vi "runTestScenario.vi"(8 "error in (no error)":errorcluster, 11 "SM_CW High Test in":refnum<class "SM_CW High Test.lvclass">) -> (0 "error out":errorcluster, 2 "TestExecution":T1, 3 "SM_CW High Test out":refnum<class "SM_CW High Test.lvclass">)   [LabVIEW 2015, in "SM_CW High Test.lvclass"]
uses:
  SM_CW High Test.lvclass
  Typedefs/TestExecution.ctl
  SM_CW High Test.lvclass/SM_CW High Test.ctl
  <userlib>/Common/ILC/Typedefs/DigitalOutputValues.ctl
  Typedefs/WriteLogMessageInput.ctl
  Typedefs/TestScenarioTypes.ctl
  Typedefs/PassFailTest.ctl
  Model/TestLog/ITestLog/ITestLog.lvclass
  Typedefs/ILCBTTypedefs.lvlib
  <userlib>/Common/ILC/ILC/ILC.lvclass
  <userlib>/Common/ILC/Typedefs/ILCTypedefs.lvlib
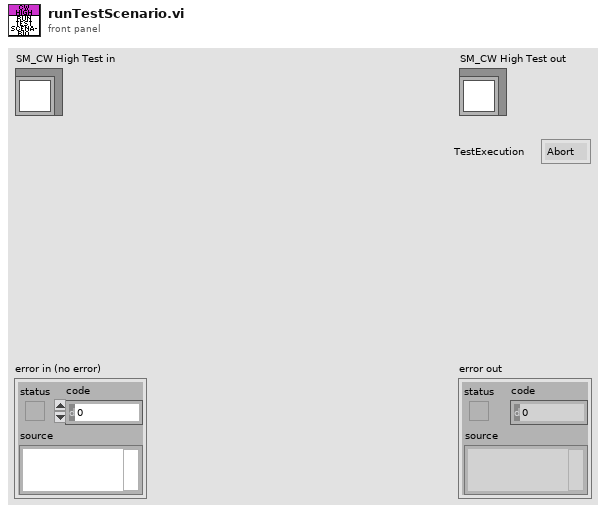
[diagram p1: front panel]
types:
  T1 = typedef "ILCBTTypedefs.lvlib/TestExecution.ctl" = enum16{"Abort", "Continue"}
  T2 = typedef "ILCBTTypedefs.lvlib/Digital Signal Level.ctl" = enum16{"Low", "High"}
  T3 = typedef "ILCBTTypedefs.lvlib/WriteLogMessageInput.ctl" = cluster{"Test Scenario":T4, "Description":string, "Actual Value":string, "Data File":string, "Result":T5}
  T4 = typedef "ILCBTTypedefs.lvlib/TestScenarioTypes.ctl" = enum16{"+3.3VA Supply Test", "+3.3VD Supply Test", "+5VA Supply Test", "+5VD Supply Test", "Unique ID Test", "TEDS Status Test", "LIMSW1_TTL Low Test", "LIMSW1_TTL High Test", "LIMSW2_TTL Low Test", "LIMSW2_TTL High Test", "Tachometer Test", "SSR_TTL Low Test", "SSR_TTL High Test", "SM_CW Low Test", "SM_CW High Test", "SM_CCW Low Test", "SM_CCW High Test", "SM_GPI Low Test", "SM_GPI High Test", "CW Motion Without Limit Test", "CW Motion With Limit Test", "CW Motion With Limit Interruption Test", "CW Motion on CCW Limit Test", "CCW Motion Without Limit Test", "CCW Motion With Limit Test", "CCW Motion With Limit Interruption Test", "CCW Motion on CW Limit Test", "RS232-TXD Low Test", "RS232-TXD High Test", "RS232-RTS Low Test", "RS232-RTS High Test", "RS232-RXD Low Test", "RS232-RXD High Test", "RS232-CTS Low Test", "RS232-CTS High Test", "Out_SS Low Test", "Out_SS High Test", "Out_SDI Low Test", "Out_SDI High Test", "Out_SCLK Low Test", "Out_SCLK High Test", "Reset Low Test", "Reset High Test", "1 Channel ADC Test", "3 Channel ADC Test", "5 Channel ADC Test", "Vref Test", "ROT Test", "DAC1 Test", "DAC2 Test", "DAC3 Test", "DAC4 Test", "BIAS Test", "EXC1 Test", "EXC2 Test", "EXC3 Test", "EXC4 Test"}
  T5 = typedef "ILCBTTypedefs.lvlib/PassFailTest.ctl" = enum16{"Fail", "Pass", "NA"}
  T6 = typedef "ILCCommon.lvlib/ILCTypedefs.lvlib/DigitalOutputValues.ctl" = cluster{"All Off":bool, "SM_CW":bool, "SM_CCW":bool, "UART2_TXD":bool, "UART2_RTS":bool, "UART2_RXD":bool, "UART2_CTS":bool, "OUT_SDO":bool, "OUT_SDI":bool, "OUT_SCK":bool, "MB_SS":bool, "MB_RESET":bool, "SSR_OUT":bool}
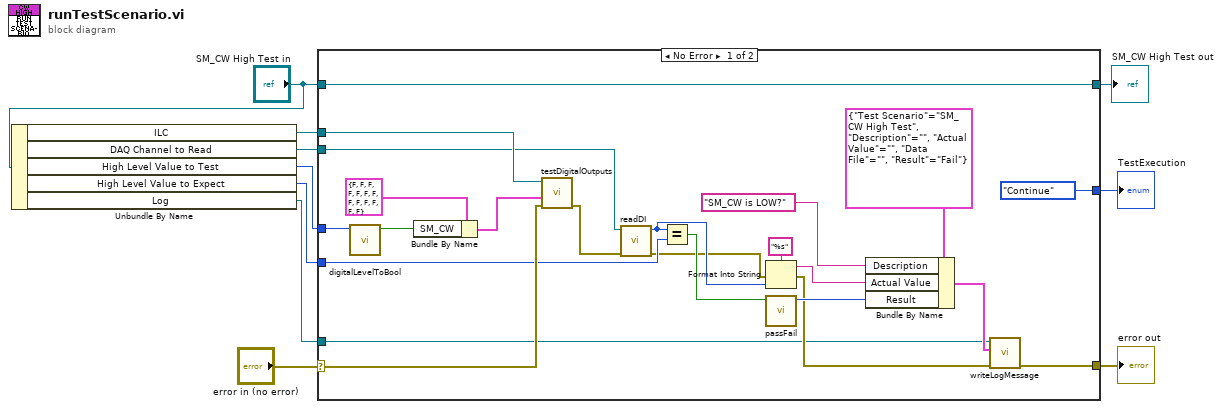
[diagram p0: block diagram]
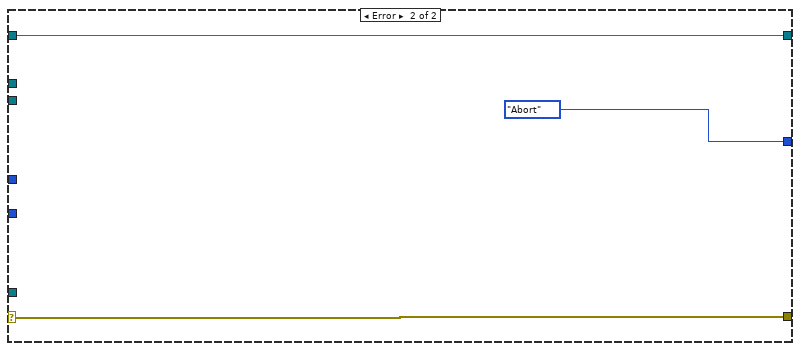
[diagram p2: hidden frame]
diagram:
  n1 = Unbundle By Name("SM_CW High Test in") -> ("ILC"=w4:refnum<class "ILC.lvclass">, "DAQ Channel to Read"=w3:refnum<k21>, "High Level Value to Test"=w5:T2, "High Level Value to Expect"=w2:T2, "Log"=w1:refnum<class "ITestLog.lvclass">)
  n2 = case shown="No Error" "error in (no error)" {
    selector: "error in (no error)" -> [w32 w35]
    tunnel: [w13 w35] -> w9
    tunnel: [w30 w36] -> w8
    tunnel: "SM_CW High Test in" -> [w30 w36]
    tunnel: [TestExecution."Continue" ("TestExecution") TestExecution."Abort" ("TestExecution")] -> w7
    tunnel: w5 -> [w27 _]
    tunnel: w4 -> [w26 _]
    tunnel: w3 -> [w24 _]
    tunnel: w2 -> [w23 _]
    tunnel: w1 -> [w11 _]
    frame No Error {
      n3 = call "digitalLevelToBool.vi"("Digital Signal Level"=w27) -> ("Bool?"=w28:bool)  [unwired: 10 in]
      n4 = Bundle By Name(cluster=T6 {"All Off"=FALSE, "SM_CW"=FALSE, "SM_CCW"=FALSE, "UART2_TXD"=FALSE, "UART2_RTS"=FALSE, "UART2_RXD"=FALSE, "UART2_CTS"=FALSE, "OUT_SDO"=FALSE, "OUT_SDI"=FALSE, "OUT_SCK"=FALSE, "MB_SS"=FALSE, "MB_RESET"=FALSE, "SSR_OUT"=FALSE} ("Digital Output Values"), "SM_CW"=w28) -> (w25:T6)
      n5 = call <userlib>:"testDigitalOutputs.vi"("error in (no error)"=w32, "Digital Output Values"=w25, "ILC in"=w26) -> ("error out"=w31:errorcluster)  [unwired: 7 in, 1 out]
      n6 = call "readDI.vi"("error in (no error)"=w31, "DAQ Channel To Read"=w24) -> ("error out"=w12:errorcluster, "Digital Signal Level"=w19:T2)  [unwired: 8 in]
      n7 = Equal?(x=w19, y=w23) -> (x = y?=w20:bool)
      n8 = Format Into String(format string="%s", error in=w12, w19) -> (resulting string=w17:string, error out=w14:errorcluster)  [unwired: 1 in]
      n9 = call "passFail.vi"("Boolean"=w20) -> ("Result"=w21:T5)  [unwired: 10 in]
      n10 = Bundle By Name(cluster=T3 {"Test Scenario"=enum."SM_CW High Test", "Description"="", "Actual Value"="", "Data File"="", "Result"=enum."Fail"} ("WriteLogMessageInput"), "Description"="SM_CW is LOW?", "Actual Value"=w17, "Result"=w21) -> (w15:T3)
      n11 = call-dynamic "writeLogMessage.vi"("error in (no error)"=w14, "WriteLogMessageInput"=w15, "ITestLog in"=w11) -> ("error out"=w13:errorcluster)  [unwired: 7 in, 1 out]
    }
    frame Error {
    }
  }
  "error out" <- w9
  "SM_CW High Test out" <- w8
  "TestExecution" <- w7
